vi "引导.vi"() -> ()   [LabVIEW 2012]
panel:
  in  "停止按钮":bool
  in  "高速采集卡实测信号仿真":bool
  in  "本地数字信号仿真":bool
  in  "本地模拟信号仿真":bool
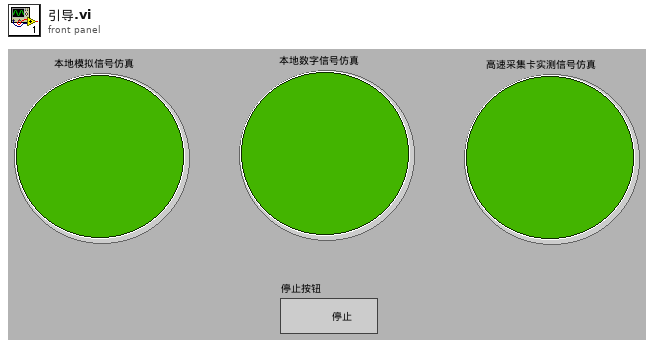
[diagram p1: front panel]
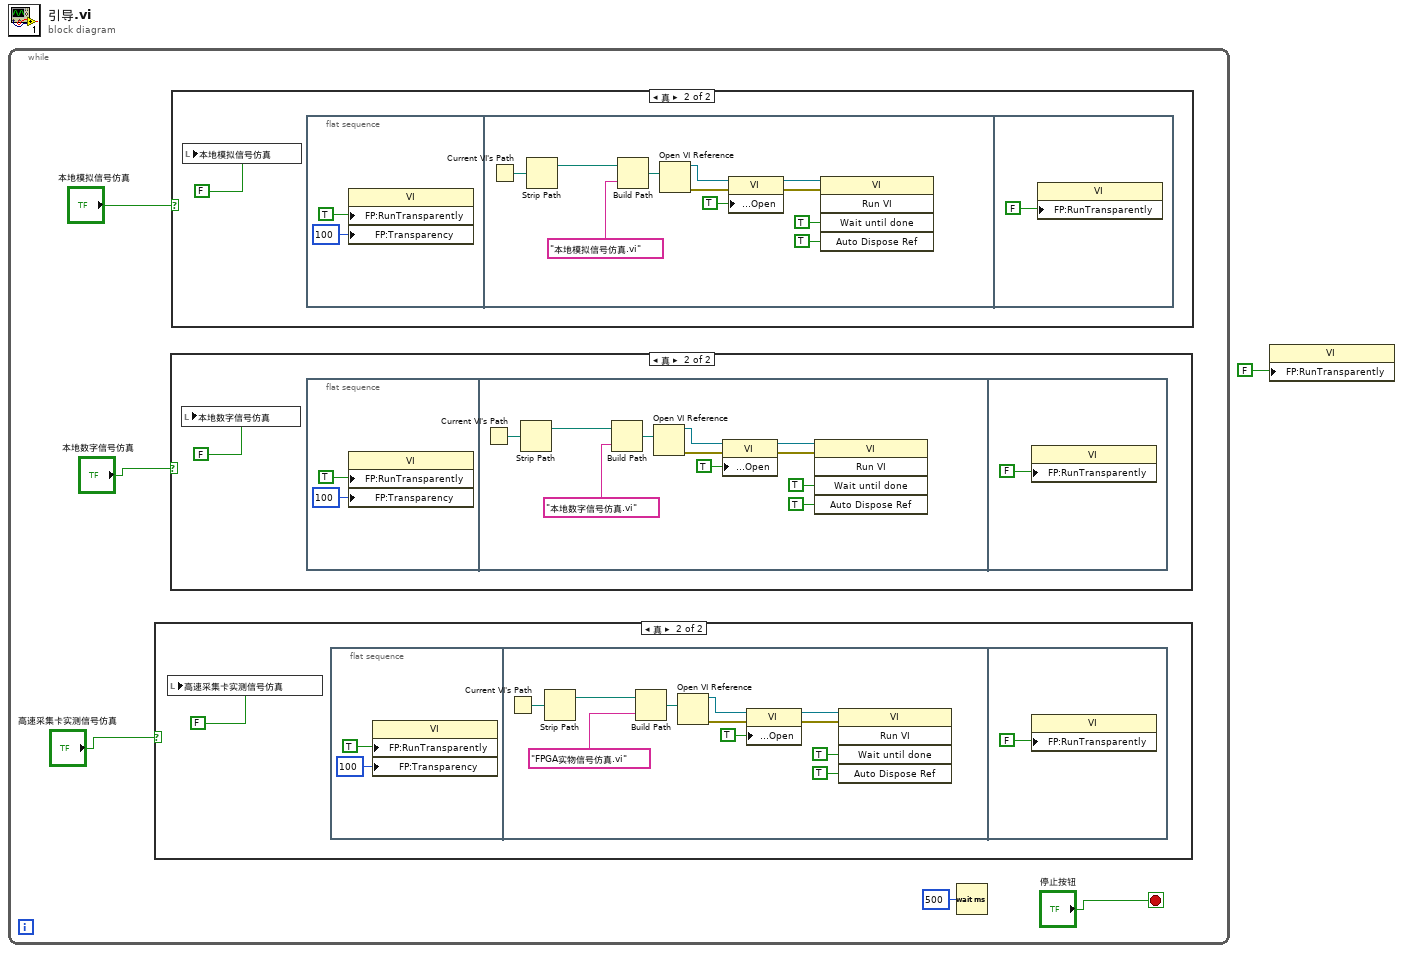
[diagram p0: block diagram]
diagram:
  n1 = while {
    stop <- "停止按钮" stop-if-true
    n2 = case shown="真" "高速采集卡实测信号仿真" {
      frame False {
      }
      frame True {
        n3 = local write "高速采集卡实测信号仿真"(FALSE ("布尔")) -> ()
        n4 = flat-sequence {
          frame #0 {
            n5 = property class="VI"("FP:RunTransparently"=TRUE ("前面板窗口:以透明方式运行VI"), "FP:Transparency"=u8 100 ("前面板窗口:透明度")) -> ()  [unwired: 2 in, 2 out]
          }
          frame #1 {
            n6 = Current VI's Path() -> (path=w10:path)
            n7 = Strip Path(path=w10) -> (stripped path=w20:path)  [unwired: 1 out]
            n8 = Build Path(base path=w20, name or relative path="FPGA实物信号仿真.vi" ("名称或相对路径")) -> (appended path=w19:path)
            n9 = Open VI Reference(vi path=w19) -> (vi reference=w18:refnum<vi>, error out=w17:errorcluster)  [unwired: 5 in]
            n10 = property class="VI"(reference=w18, error in=w17, "Front Panel.Open"=TRUE ("前面板窗口:打开")) -> (reference out=w15:refnum<vi>, error out=w14:errorcluster)
            n11 = invoke class="VI" method="Run VI"(reference=w15, error in=w14, "Wait until done"=TRUE ("结束前等待"), "Auto Dispose Ref"=TRUE ("自动销毁引用")) -> ()  [unwired: 1 in, 5 out]
          }
          frame #2 {
            n12 = property class="VI"("FP:RunTransparently"=FALSE ("前面板窗口:以透明方式运行VI")) -> ()  [unwired: 2 in, 2 out]
          }
        }
      }
    }
    n13 = case shown="真" "本地数字信号仿真" {
      frame False {
      }
      frame True {
        n14 = local write "本地数字信号仿真"(FALSE ("布尔")) -> ()
        n15 = flat-sequence {
          frame #0 {
            n16 = property class="VI"("FP:RunTransparently"=TRUE ("前面板窗口:以透明方式运行VI"), "FP:Transparency"=u8 100 ("前面板窗口:透明度")) -> ()  [unwired: 2 in, 2 out]
          }
          frame #1 {
            n17 = Current VI's Path() -> (path=w25:path)
            n18 = Strip Path(path=w25) -> (stripped path=w35:path)  [unwired: 1 out]
            n19 = Build Path(base path=w35, name or relative path="本地数字信号仿真.vi" ("名称或相对路径")) -> (appended path=w34:path)
            n20 = Open VI Reference(vi path=w34) -> (vi reference=w33:refnum<vi>, error out=w32:errorcluster)  [unwired: 5 in]
            n21 = property class="VI"(reference=w33, error in=w32, "Front Panel.Open"=TRUE ("前面板窗口:打开")) -> (reference out=w30:refnum<vi>, error out=w29:errorcluster)
            n22 = invoke class="VI" method="Run VI"(reference=w30, error in=w29, "Wait until done"=TRUE ("结束前等待"), "Auto Dispose Ref"=TRUE ("自动销毁引用")) -> ()  [unwired: 1 in, 5 out]
          }
          frame #2 {
            n23 = property class="VI"("FP:RunTransparently"=FALSE ("前面板窗口:以透明方式运行VI")) -> ()  [unwired: 2 in, 2 out]
          }
        }
      }
    }
    n24 = case shown="真" "本地模拟信号仿真" {
      frame False {
      }
      frame True {
        n25 = local write "本地模拟信号仿真"(FALSE ("布尔")) -> ()
        n26 = flat-sequence {
          frame #0 {
            n27 = property class="VI"("FP:RunTransparently"=TRUE ("前面板窗口:以透明方式运行VI"), "FP:Transparency"=u8 100 ("前面板窗口:透明度")) -> ()  [unwired: 2 in, 2 out]
          }
          frame #1 {
            n28 = Current VI's Path() -> (path=w40:path)
            n29 = Strip Path(path=w40) -> (stripped path=w50:path)  [unwired: 1 out]
            n30 = Build Path(base path=w50, name or relative path="本地模拟信号仿真.vi" ("名称或相对路径")) -> (appended path=w49:path)
            n31 = Open VI Reference(vi path=w49) -> (vi reference=w48:refnum<vi>, error out=w47:errorcluster)  [unwired: 5 in]
            n32 = property class="VI"(reference=w48, error in=w47, "Front Panel.Open"=TRUE ("前面板窗口:打开")) -> (reference out=w45:refnum<vi>, error out=w44:errorcluster)
            n33 = invoke class="VI" method="Run VI"(reference=w45, error in=w44, "Wait until done"=TRUE ("结束前等待"), "Auto Dispose Ref"=TRUE ("自动销毁引用")) -> ()  [unwired: 1 in, 5 out]
          }
          frame #2 {
            n34 = property class="VI"("FP:RunTransparently"=FALSE ("前面板窗口:以透明方式运行VI")) -> ()  [unwired: 2 in, 2 out]
          }
        }
      }
    }
    n35 = Wait (ms)(milliseconds to wait=u32 500 ("等待时间（毫秒）")) -> ()  [unwired: 1 out]
  }
  n36 = property class="VI"("FP:RunTransparently"=FALSE ("前面板窗口:以透明方式运行VI")) -> ()  [unwired: 2 in, 2 out]
